vi "PulseTrainGenerator-Single.vi"(8 "Stop Button":bool) -> ()   [LabVIEW 2015]
panel:
  in  "Ch Setup":T1={"IP Address"="192.168.126.147", "DIO #"=0, "Frequency (Hz)"=100.0, "duty cycle (%)"=0.5, "Enable"=FALSE} {"duty cycle (%)" min=0.01 max=0.99 step=0.1; "Frequency (Hz)" min=0.0 step=10.0}
  in  "Startup Index":u16
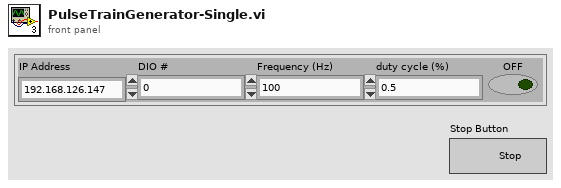
[diagram p1: front panel]
types:
  T1 = cluster{"IP Address":string, "DIO #":u16, "Frequency (Hz)":dbl, "duty cycle (%)":dbl, "Enable":bool}
  T2 = enum16{"Enable", "Disable", "Change Frequency", "Change Duty Cycle", "Configure", "Configure and Run"}
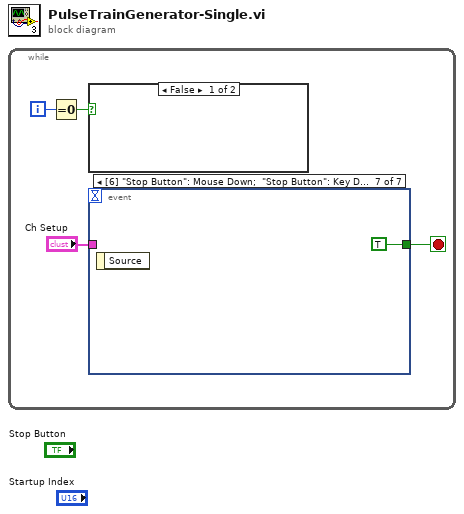
[diagram p0: block diagram]
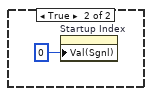
[diagram p2: hidden frame]
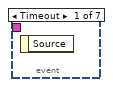
[diagram p3: hidden frame]
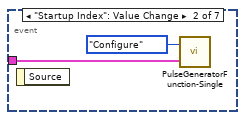
[diagram p4: hidden frame]
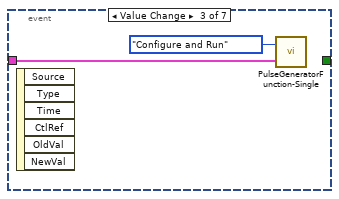
[diagram p5: hidden frame]
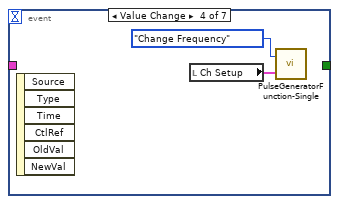
[diagram p6: hidden frame]
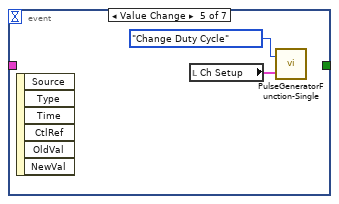
[diagram p7: hidden frame]
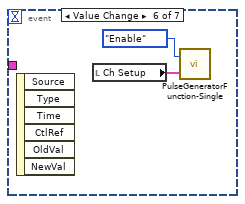
[diagram p8: hidden frame]
diagram:
  n1 = while {
    i -> [w4]
    stop <- w2 stop-if-true
    n2 = Equal To 0?(x=w4) -> (x = 0?=w3:bool)
    n3 = case shown="False" w3 {
      frame False {
      }
      frame True {
        n4 = property on="Startup Index" class="DigNum (strict)"("Val(Sgnl)"=u16 0 ("Value (Signaling)")) -> ()  [unwired: 2 in, 2 out]
      }
    }
    n5 = event shown="[6] \"Stop Button\": Mouse Down;  \"Stop Button\": Key Down" {
      selector: _ -> [_ _ _ _ _ _ _]
      dyn-events: _ -> [_ _ _ _ _ _ _]
      timeout: _ -> [_ _ _ _ _ _ _]
      tunnel: "Ch Setup" -> [_ w7 w9 _ _ _ _]
      tunnel: [_ _ _ _ _ _ TRUE] -> w2
      event Timeout {
        n6 = event-data() -> ()  [unwired: 1 in, 1 out]
      }
      event "Startup Index": Value Change {
        n7 = event-data() -> ()  [unwired: 1 in, 1 out]
        n8 = call "PulseGeneratorFunction-Single.vi"("Ch Setup"=w7, "Mode"=T2."Configure") -> ()  [unwired: 1 in]
      }
      event "Ch Setup.IP Address", "Ch Setup.DIO #": Value Change {
        n9 = event-data() -> ()  [unwired: 1 in, 6 out]
        n10 = call "PulseGeneratorFunction-Single.vi"("Ch Setup"=w9, "Mode"=T2."Configure and Run") -> ()  [unwired: 1 in]
      }
      event "Ch Setup.Frequency (Hz)": Value Change {
        n11 = event-data() -> ()  [unwired: 1 in, 6 out]
        n12 = local read "Ch Setup"() -> (w11:T1)
        n13 = call "PulseGeneratorFunction-Single.vi"("Ch Setup"=w11, "Mode"=T2."Change Frequency") -> ()  [unwired: 1 in]
      }
      event "Ch Setup.duty cycle (%)": Value Change {
        n14 = event-data() -> ()  [unwired: 1 in, 6 out]
        n15 = local read "Ch Setup"() -> (w13:T1)
        n16 = call "PulseGeneratorFunction-Single.vi"("Ch Setup"=w13, "Mode"=T2."Change Duty Cycle") -> ()  [unwired: 1 in]
      }
      event "Ch Setup.Enable": Value Change {
        n17 = event-data() -> ()  [unwired: 1 in, 6 out]
        n18 = local read "Ch Setup"() -> (w15:T1)
        n19 = call "PulseGeneratorFunction-Single.vi"("Ch Setup"=w15, "Mode"=T2."Enable") -> ()  [unwired: 1 in]
      }
      event "Stop Button": Mouse Down; "Stop Button": Key Down {
        n20 = event-data() -> ()  [unwired: 1 in, 1 out]
      }
    }
  }
